vi "Run Data.vi"(4 "Params 2D IN":variant[][](array[variant]), 5 "Param Names IN":string[](array[string]), 6 "Params 1D IN":variant[](array[variant]), 7 "Index Number":i32, 8 "error in":errorcluster, 9 "Data 2D IN":dbl[][](array[numeric]), 10 "Data 1D IN":dbl[](array[numeric]), 11 "action":T1) -> (0 "error out":errorcluster, 1 "Param Names OUT":string[](array[string]), 2 "Params 1D OUT":variant[](array[variant]), 3 "Data 1D OUT":dbl[](array[numeric]))   [LabVIEW 2011]
uses:
  Run Data.ctl
  <vilib>/Analysis/NI_AALBase.lvlib
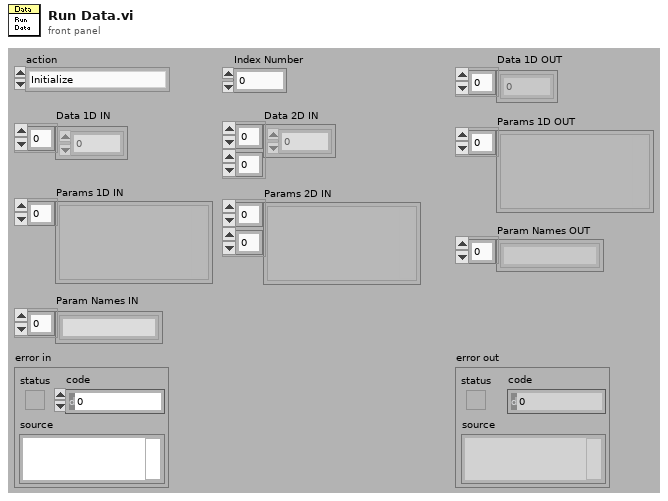
[diagram p1: front panel]
types:
  T1 = typedef "Run Data.ctl" = enum16{"Initialize", "Add Sample Channel", "Set Run", "Get Number of Runs", "Set Run Params", "Get Spectrum", "Get Run Params", "Get Sample Params", "Get History", "Get Averaged History", "Get Run Param Names", "Set Run Param Names", "Get Sample Param Names", "Set Sample Param Names", "Get MFC Flow Rate Challenge Profile", "Get History Average"}
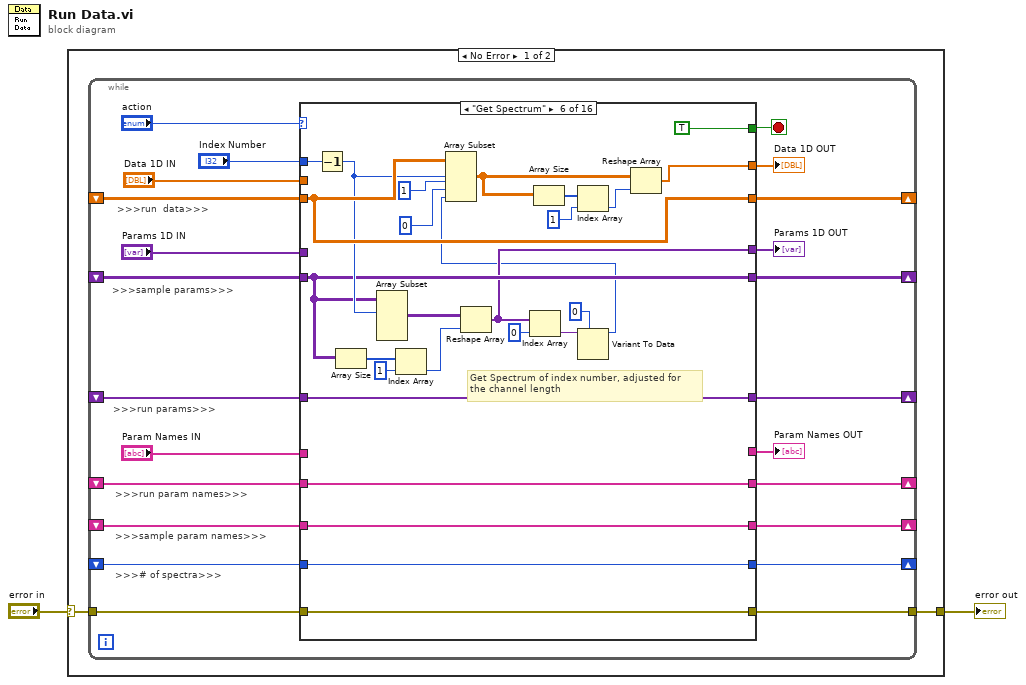
[diagram p0: block diagram]
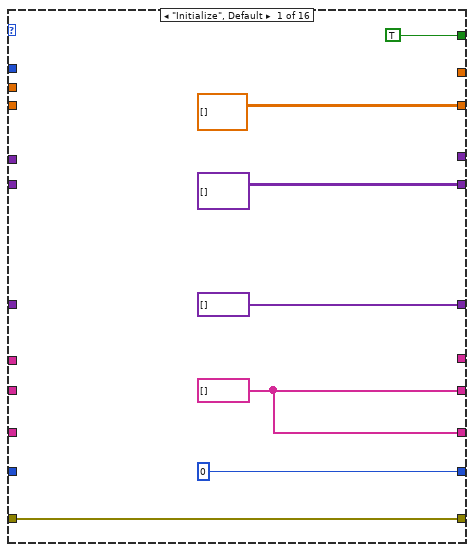
[diagram p2: hidden frame]
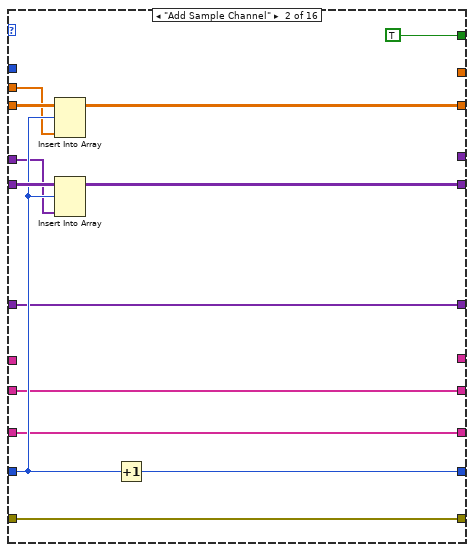
[diagram p3: hidden frame]
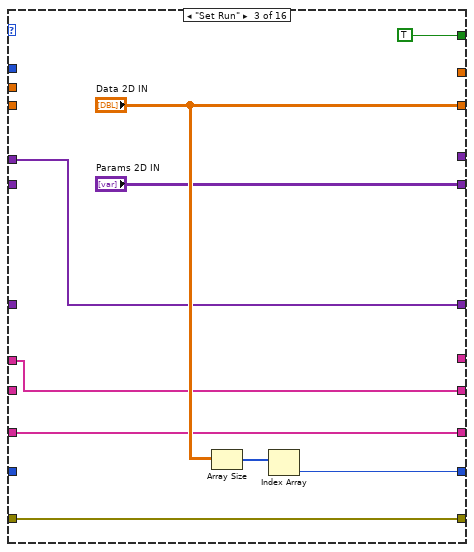
[diagram p4: hidden frame]
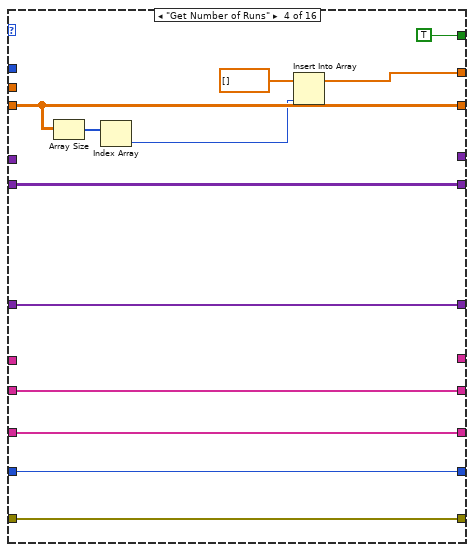
[diagram p5: hidden frame]
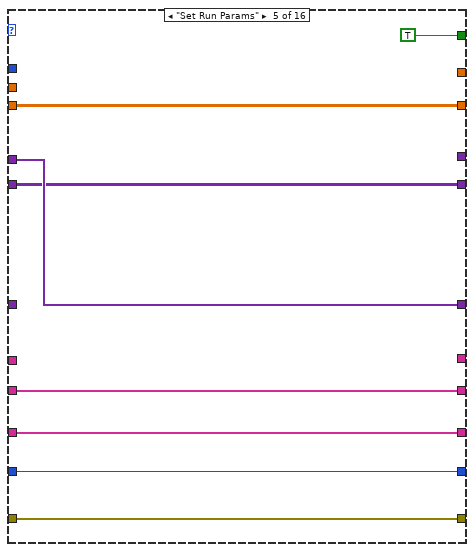
[diagram p6: hidden frame]
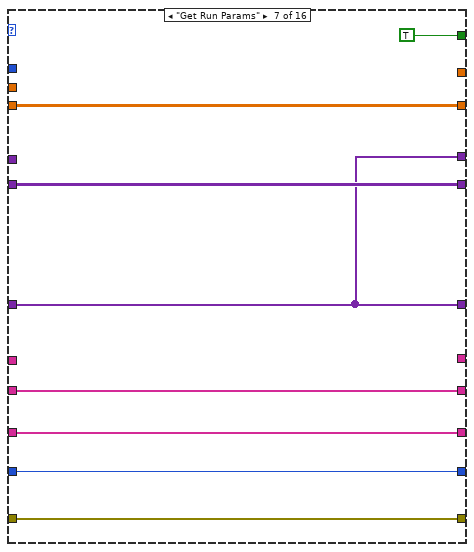
[diagram p7: hidden frame]
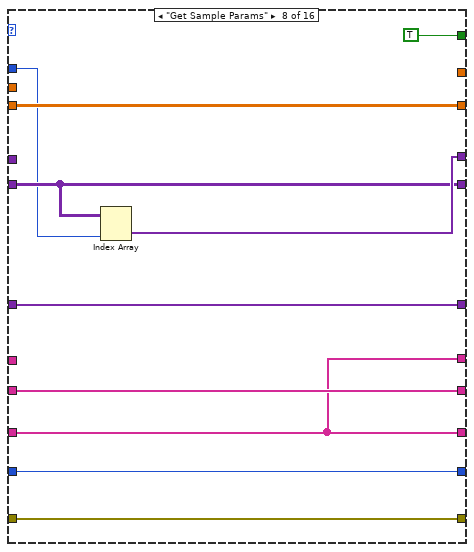
[diagram p8: hidden frame]
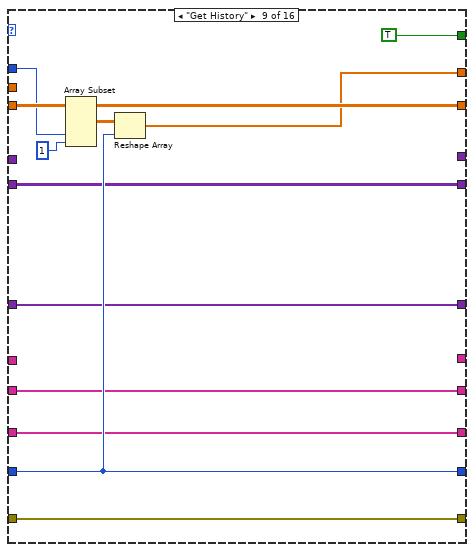
[diagram p9: hidden frame]
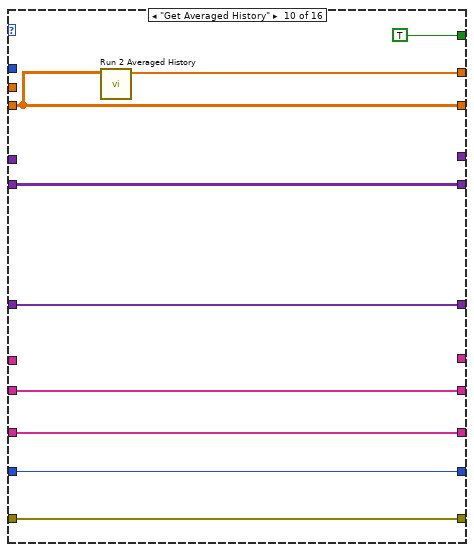
[diagram p10: hidden frame]
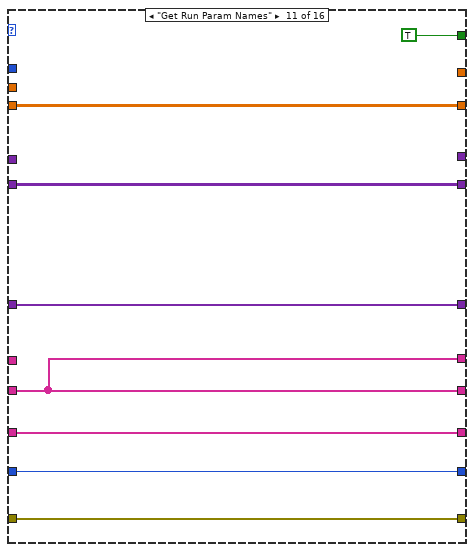
[diagram p11: hidden frame]
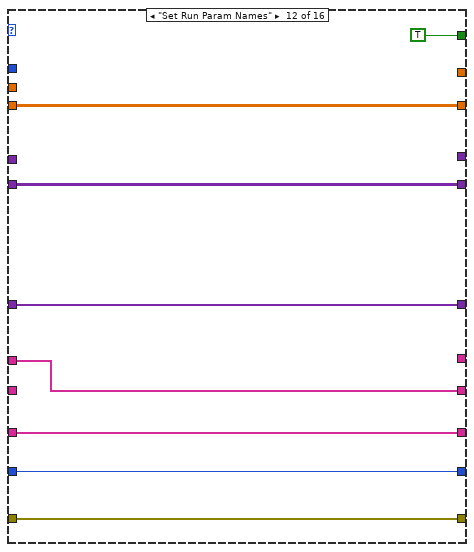
[diagram p12: hidden frame]
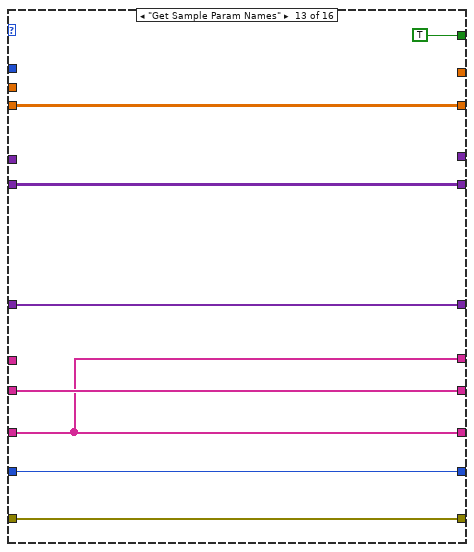
[diagram p13: hidden frame]
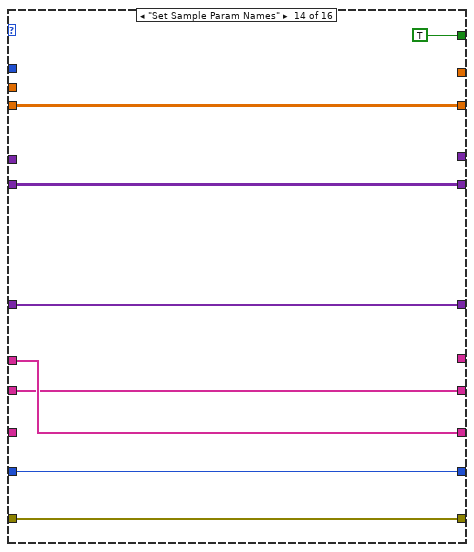
[diagram p14: hidden frame]
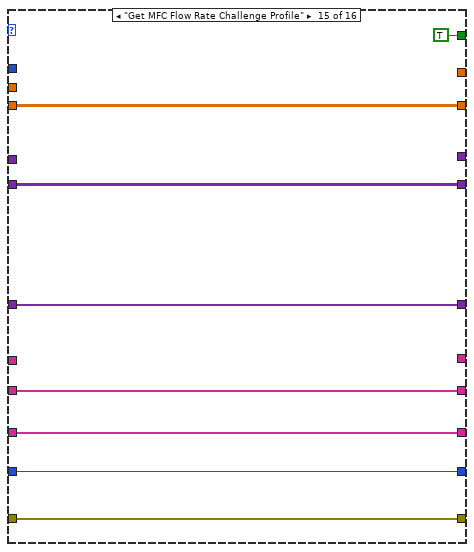
[diagram p15: hidden frame]
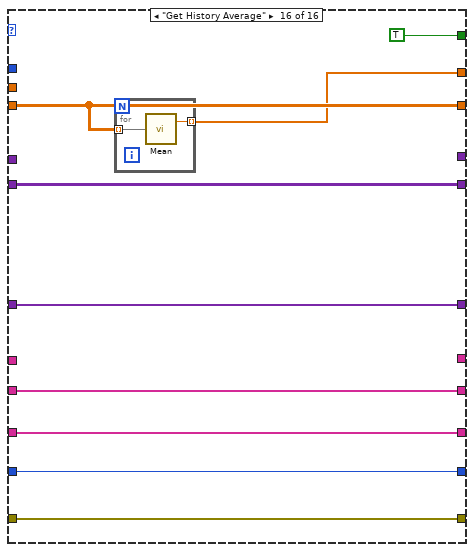
[diagram p16: hidden frame]
diagram:
  n1 = case shown="No Error" "error in" {
    selector: "error in" -> [w4 w193]
    tunnel: [w3 w193] -> w1
    frame No Error {
      n2 = while {
        shift-right: [w26] -> _
        shift-left: _ -> [w25]
        shift-right: [w24] -> _
        shift-left: _ -> [w23]
        tunnel: w4 -> [w22]
        tunnel: [w21] -> w3
        shift-right: [w19] -> _
        shift-left: _ -> [w18]
        shift-right: [w17] -> _
        shift-left: _ -> [w16]
        shift-right: [w13] -> _
        shift-left: _ -> [w11]
        shift-right: [w12] -> _
        shift-left: _ -> [w10]
        stop <- w20 stop-if-true
        # ">>>sample param names>>>"
        # ">>>run param names>>>"
        # ">>>run params>>>"
        # ">>># of spectra>>>"
        # ">>>sample params>>>"
        # ">>>run  data>>>"
        n3 = case shown="\"Get Spectrum\"" "action" {
          tunnel: [dbl[][] [] w45 "Data 2D IN" w67 w75 w96 w110 w120 w131 w133 w148 w156 w165 w167 w181 w186] -> w26
          tunnel: w25 -> [_ w47 _ w67 w75 w96 w110 w120 w131 w133 w148 w156 w165 w167 w181 w186]
          tunnel: [0 w46 w52 w61 w70 w100 w107 w117 w127 w137 w143 w152 w159 w171 w177 w188] -> w24
          tunnel: w23 -> [_ w41 _ w61 w70 w100 w107 w117 w127 w137 w143 w152 w159 w171 w177 w188]
          tunnel: w22 -> [w32 w44 w55 w60 w69 w101 w106 w118 w130 w136 w142 w151 w158 w170 w175 w187]
          tunnel: [w32 w44 w55 w60 w69 w101 w106 w118 w130 w136 w142 w151 w158 w170 w175 w187] -> w21
          tunnel: [TRUE TRUE TRUE TRUE TRUE TRUE TRUE TRUE TRUE TRUE TRUE TRUE TRUE TRUE TRUE TRUE] -> w20
          tunnel: [variant[][] [] ("values") w40 "Params 2D IN" w65 w73 w94 w108 w115 w126 w141 w147 w155 w163 w168 w176 w189] -> w19
          tunnel: w18 -> [_ w42 _ w65 w73 w94 w108 w115 w126 w141 w147 w155 w163 w168 w176 w189]
          tunnel: [_ _ _ w57 _ w77 _ _ w125 w134 _ _ _ _ _ w185] -> w6
          tunnel: [variant[] [] ("Params 1D IN") w39 w50 w64 w74 w93 w103 w119 w124 w140 w146 w150 w162 w169 w180 w184] -> w17
          tunnel: w16 -> [_ w39 _ w64 _ w93 w103 w119 w124 w140 w146 w150 w162 w169 w180 w184]
          tunnel: "Params 1D IN" -> [_ w36 w50 _ w74 _ _ _ _ _ _ _ _ _ _ _]
          tunnel: "Param Names IN" -> [_ _ w48 _ _ _ _ _ _ _ _ w154 _ w173 _ _]
          tunnel: [w29 w38 w48 w63 w72 w92 w105 w113 w123 w139 w145 w154 w161 w172 w178 w183] -> w13
          tunnel: [w29 w37 w49 w62 w71 w91 w104 w112 w122 w138 w144 w153 w160 w173 w179 w182] -> w12
          tunnel: w11 -> [_ w38 _ w63 w72 w92 w105 w113 w123 w139 w145 _ w161 w172 w178 w183]
          tunnel: w10 -> [_ w37 w49 w62 w71 w91 w104 w112 w122 w138 w144 w153 w160 _ w179 w182]
          tunnel: [_ _ _ _ _ _ _ w112 _ _ w145 _ w160 _ _ _] -> w9
          tunnel: [_ _ _ _ _ w89 w103 w116 _ _ _ _ _ _ _ _] -> w8
          tunnel: "Data 1D IN" -> [_ w35 _ _ _ _ _ _ _ _ _ _ _ _ _ _]
          tunnel: "Index Number" -> [_ _ _ _ _ w90 _ w111 w121 _ _ _ _ _ _ _]
          frame "Initialize", Default {
            w29 = string[] [] ("Param Names IN")
          }
          frame "Add Sample Channel" {
            n4 = Insert Into Array(array=w47, index (row)=w41, new element=w35) -> (w45:dbl[][])  [unwired: 1 in]
            n5 = Insert Into Array(array=w42, index (row)=w41, new element=w36) -> (w40:variant[][])  [unwired: 1 in]
            n6 = Increment(x=w41) -> (x+1=w46:i32)
          }
          frame "Set Run" {
            n7 = Array Size(array="Data 2D IN") -> (size(s)=w53:i32[])
            n8 = Index Array(array=w53) -> (element=w52:i32)  [unwired: 1 in]
          }
          frame "Get Number of Runs" {
            n9 = Array Size(array=w67) -> (size(s)=w66:i32[])
            n10 = Index Array(array=w66) -> (element=w58:i32)  [unwired: 1 in]
            n11 = Insert Into Array(array=dbl[] [], new element=w58) -> (w57:dbl[])  [unwired: 1 in]
          }
          frame "Set Run Params" {
          }
          frame "Get Spectrum" {
            # "Get Spectrum of index number, adjusted for\nthe channel length"
            n12 = Decrement(x=w90) -> (x-1=w95:i32)
            n13 = Array Size(array=w94) -> (size(s)=w98:i32[])
            n14 = Array Subset(array=w94, index (row)=w95) -> (w99:variant[][])  [unwired: 3 in]
            n15 = Index Array(array=w98, index=1) -> (element=w85:i32)
            n16 = Reshape Array(w99, w85) -> (w89:variant[])
            n17 = Index Array(array=w89, index=0) -> (element=w87:variant)
            n18 = Variant To Data(type=0 ("index"), Variant=w87) -> (data=w82:i32)  [unwired: 1 in, 1 out]
            n19 = Array Subset(array=w96, index (row)=w95, length (row)=1 ("length"), index (col)=0 ("index"), length (col)=w82) -> (w79:dbl[][])
            n20 = Array Size(array=w79) -> (size(s)=w81:i32[])
            n21 = Index Array(array=w81, index=1) -> (element=w78:i32)
            n22 = Reshape Array(w79, w78) -> (w77:dbl[])
          }
          frame "Get Run Params" {
          }
          frame "Get Sample Params" {
            n23 = Index Array(array=w115, index (col)=w111) -> (element=w116:variant[])  [unwired: 1 in]
          }
          frame "Get History" {
            n24 = Array Subset(array=w131, index (col)=w121, length (col)=1 ("length")) -> (w132:dbl[][])  [unwired: 2 in]
            n25 = Reshape Array(w132, w127) -> (w125:dbl[])
          }
          frame "Get Averaged History" {
            n26 = call "Run 2 Averaged History.vi"("2D Run Data"=w133) -> ("Data 2D IN out"=w134:dbl[])  [unwired: 10 in]
          }
          frame "Get Run Param Names" {
          }
          frame "Set Run Param Names" {
          }
          frame "Get Sample Param Names" {
          }
          frame "Set Sample Param Names" {
          }
          frame "Get MFC Flow Rate Challenge Profile" {
          }
          frame "Get History Average" {
            n27 = for {
              tunnel: w186 -> [w192] mode=indexing
              tunnel: [w191] -> w185 mode=indexing
              n28 = call <vilib>:"Mean.vi"("X"=w192) -> ("mean"=w191:dbl)  [unwired: 1 out]
            }
          }
        }
        "Param Names OUT" <- w9
        "Params 1D OUT" <- w8
        "Data 1D OUT" <- w6
      }
    }
    frame Error {
    }
  }
  "error out" <- w1
